vi "Process Read.vi"(8 "error in (no error)":errorcluster, 10 "gRPCid":T1, 11 "Data Server":refnum<class "Data Server.lvclass">) -> (0 "error out":errorcluster)   [LabVIEW 2020, in "Veristandgrpc_server.lvlib" / "veristand-grpc.lvclass"]
uses:
  veristand-grpc.lvclass
  Data/Data Server.lvclass
  <vilib>/gRPC/LabVIEW gRPC Library/Shared/grpcId.ctl
  RPC Messages/veristand_Reponse.ctl
  Data/Data Server.lvclass/Data Server.ctl
  Veristandgrpc_server.lvlib
  <vilib>/gRPC/LabVIEW gRPC Library/grpc-lvsupport-release.lvlib
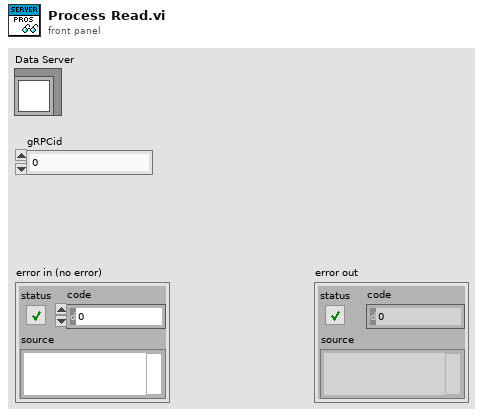
[diagram p1: front panel]
types:
  T1 = typedef "grpc-lvsupport-release.lvlib/grpcId.ctl" = u64
  T2 = typedef "Veristandgrpc_server.lvlib/veristand_Reponse.ctl" = cluster{"status":string, "data":string}
  T3 = typedef "Veristandgrpc_server.lvlib/veristand_Request.ctl" = cluster{"server":string, "channel":string, "data":string}
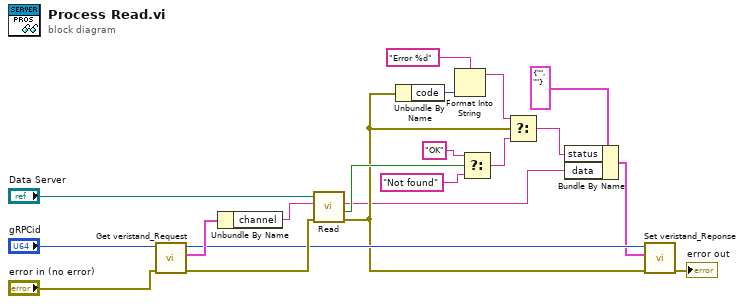
[diagram p0: block diagram]
diagram:
  n1 = call "Get veristand_Request.vi"("error in (no error)"="error in (no error)", "gRPCid"="gRPCid") -> ("error out"=w16:errorcluster, "package_templatemessage"=w18:T3, "gRPCid out"=w6:T1)  [unwired: 7 in]
  n2 = Unbundle By Name(w18) -> ("channel"=w2:string)
  n3 = call "Read.vi"("error in (no error)"=w16, "Channel Name"=w2, "Data in"="Data Server") -> ("error out"=w5:errorcluster, "Found"=w7:bool, "Data"=w1:string)  [unwired: 5 in, 1 out]
  n4 = Unbundle By Name(w5) -> ("code"=w13:i32)
  n5 = Format Into String(format string="Error %d", w13) -> (resulting string=w14:string)  [unwired: 2 in, 1 out]
  n6 = Select(t="OK" ("data"), s=w7, f="Not found" ("data")) -> (s? t:f=w9:string)
  n7 = Select(t=w14, s=w5, f=w9) -> (s? t:f=w15:string)
  n8 = Bundle By Name(cluster=T2 {"status"="", "data"=""} ("veristand_Reponse"), "status"=w15, "data"=w1) -> (w4:T2)
  n9 = call "Set veristand_Reponse.vi"("error in (no error)"=w5, "package_templatemessage"=w4, "gRPCid"=w6) -> ("error out"=→"error out":errorcluster)  [unwired: 8 in]
